vi "Parallel - Threaded.vi"(10 "Status Calculation":T1, 11 "Nodes":refnum<class "bt_Node.lvclass">[](array[class])) -> (3 "Node":refnum<class "bt_Node.lvclass">)   [LabVIEW 2021, in "BT.lvlib"]
uses:
  BT.lvlib
  Support/Nodes/Composites/Parallel_Threaded/bt_Parallel_Threaded.lvclass
  C:/Users/Tim/Documents/GitHub/LV_Behaviour_Tree/Source/Support/Nodes/abs_Node/bt_Node.lvclass
  Support/Nodes/abs_Node/bt_Node.lvclass
  Support/Nodes/Composites/abs_Parallel/Support/Status Calculation.ctl
  Support/Nodes/Composites/abs_Parallel/bt_Parallel.lvclass
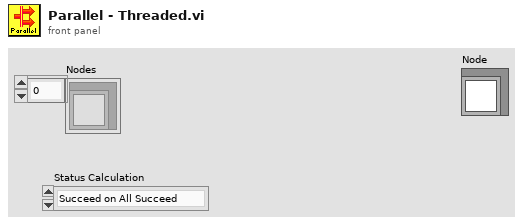
[diagram p1: front panel]
types:
  T1 = typedef "BT.lvlib/bt_Parallel.lvclass/Status Calculation.ctl" = enum16{"Succeed on All Succeed", "Failure on All Failure", "Succeed on Any Succeed", "Failure on Any Failure"}
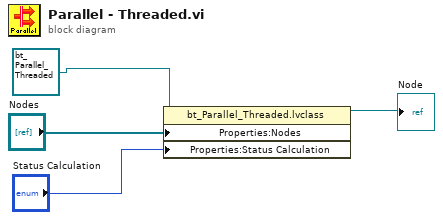
[diagram p0: block diagram]
diagram:
  n1 = property class="bt_Parallel_Threaded.lvclass"(reference=refnum<class "bt_Parallel_Threaded.lvclass"> refnum ("BT.lvlib:bt_Parallel_Threaded.lvclass"), "Properties:Nodes"="Nodes", "Properties:Status Calculation"="Status Calculation") -> (reference out=→"Node":refnum<class "bt_Parallel_Threaded.lvclass">)  [unwired: 1 in, 1 out]
